vi "gm_ui_meas_timetable.vi"(6 "timetable":string[][](array[string]), 7 "meas timetable":bool, 9 "measuring mode":refnum<vi>, 10 "measuring point":refnum<vi>, 11 "Boolean in":refnum<vi>) -> ()   [LabVIEW 2011]
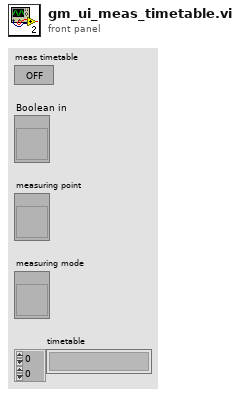
[diagram p1: front panel]
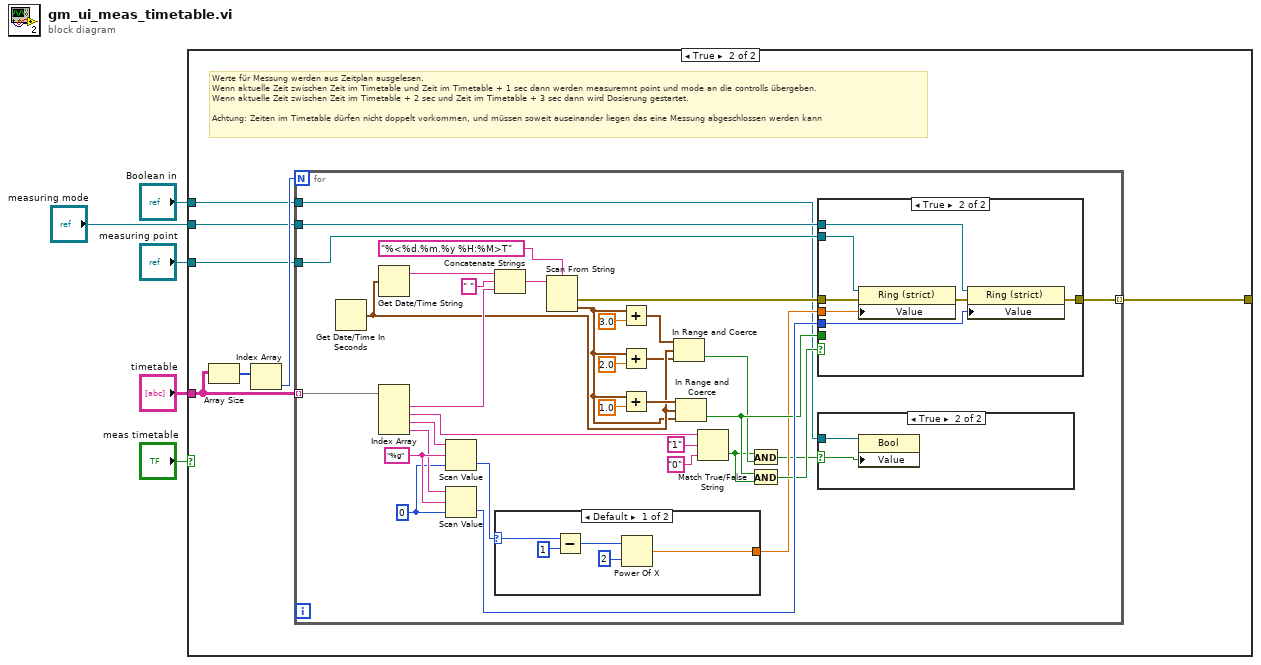
[diagram p0: block diagram]
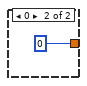
[diagram p4: hidden frame]
diagram:
  n1 = case shown="True" "meas timetable" {
    tunnel: "timetable" -> [_ w12]
    tunnel: "Boolean in" -> [_ w9]
    tunnel: "measuring point" -> [_ w8]
    tunnel: [_ w7] -> _
    tunnel: "measuring mode" -> [_ w6]
    frame False {
    }
    frame True {
      # "Werte für Messung werden aus Zeitplan ausgelesen.\nWenn aktuelle Zeit zwischen Zeit im Timetable und Zeit im Timetable + 1 sec dann werden measuremnt point und mode an die controlls übergeben.\nWenn aktuelle Zeit zwischen Zeit im Timetable + 2 sec und Zeit im Timetable + 3 sec dann wird Dosierung gestartet.\n\nAchtung: Zeiten im Timetable dürfen nicht doppelt vorkommen, und müssen soweit auseinander liegen das eine Messung abgeschlossen werden kann"
      n2 = Array Size(array=w12) -> (size(s)=w11:i32[])
      n3 = Index Array(array=w11) -> (element=w10:i32)  [unwired: 1 in]
      n4 = for {
        N: w10 -> [_]
        tunnel: w12 -> [w46] mode=indexing
        tunnel: w9 -> [w16]
        tunnel: w8 -> [w27]
        tunnel: [w25] -> w7 mode=indexing
        tunnel: w6 -> [w24]
        w13 = u32 0 ("default (0 dbl)")
        w37 = "%g" ("format string")
        n5 = Get Date/Time In Seconds() -> (seconds since 1Jan1904=w23:timestamp)
        n6 = Get Date/Time String(seconds (now)=w23) -> (date string=w31:string)  [unwired: 2 in, 1 out]
        n7 = Index Array(array=w46) -> (element #1=w45:string, element #2=w41:string, element #3=w33:string, element #4=w32:string)  [unwired: 4 in]
        n8 = Scan Value(string=w33, format string=w37, default (0 dbl)=w13) -> (value=w28:u32)  [unwired: 1 out]
        n9 = Scan Value(string=w32, format string=w37, default (0 dbl)=w13) -> (value=w38:u32)  [unwired: 1 out]
        n10 = Concatenate Strings(w31, " " ("string"), w45) -> (w34:string)
        n11 = case shown="Default" w28 {
          selector: w28 -> [w53 _]
          tunnel: [w51 u8 0 ("Value")] -> w29
          frame Default {
            n12 = Subtract(x=w53, y=u32 1) -> (x-y=w50:u32)
            n13 = Power Of X(1:u32 2 ("x"), 2:w50) -> (0:w51:dbl)
          }
          frame 0 {
          }
        }
        n14 = Scan From String(format string="%<%d.%m.%y %H:%M>T", input string=w34) -> (error out=w26:errorcluster, output 1=w21:timestamp)  [unwired: 3 in, 2 out]
        n15 = Add(x=w21, y=3.0) -> (x+y=w22:timestamp)
        n16 = Add(x=w21, y=2.0) -> (x+y=w15:timestamp)
        n17 = Add(x=w21, y=1.0) -> (x+y=w43:timestamp)
        n18 = In Range and Coerce(upper limit=w22, x=w23, lower limit=w15) -> (In Range?=w18:bool)  [unwired: 1 out]
        n19 = In Range and Coerce(upper limit=w43, x=w23, lower limit=w21) -> (In Range?=w35:bool)  [unwired: 1 out]
        n20 = Match True/False String(2:"0" ("false string"), 3:"1" ("true string"), 4:w41) -> (0:w17:bool)  [unwired: 1 out]
        n21 = And(x=w17, y=w18) -> (x .and. y?=w19:bool)
        n22 = And(x=w35, y=w17) -> (x .and. y?=w36:bool)
        n23 = case shown="True" w36 {
          tunnel: w35 -> [_ _]
          tunnel: w38 -> [_ w56]
          tunnel: w29 -> [_ w59]
          tunnel: w27 -> [_ w60]
          tunnel: w26 -> [w55 w58]
          tunnel: [w55 w61] -> w25
          tunnel: w24 -> [_ w62]
          frame False {
          }
          frame True {
            n24 = property class="Ring (strict)"(reference=w60, error in=w58, "Value"=w59) -> (error out=w57:errorcluster)  [unwired: 1 out]
            n25 = property on="Property Node" class="Ring (strict)"(reference=w62, error in=w57, "Value"=w56) -> (error out=w61:errorcluster)  [unwired: 1 out]
          }
        }
        n26 = case shown="True" w19 {
          selector: w19 -> [_ w47]
          tunnel: w16 -> [_ w48]
          frame False {
          }
          frame True {
            n27 = property on="Property Node" class="Bool"(reference=w48, "Value"=w47) -> ()  [unwired: 1 in, 2 out]
          }
        }
      }
    }
  }
